vi "PhotonCamera_GetLatestResult.vi"(6 "EstimatedDataAndSampleLatency (Sec)":dbl=0.05 format="%#_13g", 8 "Pass_Through_Time":dbl=-1.0 format="%33.4f", 11 "CameraName":string) -> (1 "HasTargets":bool, 3 "PipelineResult":T1 {"Targets"."AltCameraToTarget"."TRANSLATION3D"."Z" format="%14.3f"; "Targets"."AltCameraToTarget"."TRANSLATION3D"."Y" format="%14.3f"; "Targets"."AltCameraToTarget"."TRANSLATION3D"."X" format="%14.3f"; "Targets"."BestCameraToTarget"."TRANSLATION3D"."Z" format="%14.3f"; "Targets"."BestCameraToTarget"."TRANSLATION3D"."Y" format="%14.3f"; "Targets"."BestCameraToTarget"."TRANSLATION3D"."X" format="%14.3f"})   [LabVIEW 2019, in "PhotonVisionLib.lvlib"]
doc: "Returns the latest pipeline result.\n\nInputs:\n - cameraName -- The nickname of the camera (found in the PhotonVision UI).\n - PassThroughTime -- (Optional. Default: Use FPGA time.) Time. Once time is available from network tables, this won't be needed. (Seconds)\n - EstimatedDataAndSampleLatency -- Estimated Network Table packet latency. This is based on the frames per second and other communications latencies. (Optional. Default: 0.050) Once time is available from network tables, this won't be needed. \n\nOutputs:\n - PipelineResult -- The latest pipeline result data cluster\n - HasTargets -- Boolean indicating if any targets were found"
uses:
  PhotonVisionLib.lvlib
  TypeDef/PhotonPipelineResultType.ctl
  TypeDef/PhotonTrackedTargetType.ctl
  TypeDef/TargetCornerType.ctl
  <vilib>/Rock Robotics/WPI/ThirdParty/JAS_Junk/TrajLib/TypeDef/TRANSFORM3D.ctl
  <vilib>/Rock Robotics/WPI/ThirdParty/JAS_Junk/TrajLib/TypeDef/TRANSLATION3D.ctl
  <vilib>/Rock Robotics/WPI/ThirdParty/JAS_Junk/TrajLib/TypeDef/ROTATION3D.ctl
  <vilib>/Rock Robotics/WPI/ThirdParty/JAS_Junk/TrajLib/TypeDef/QUATERNION.ctl
  Packet_decode_Flt64.vi
  Packet_decode_ByteI8.vi
  PhotonTrackedTarget_CreateFromPacket.vi
  TargetCorner_New.vi
  Packet_decode_Int32.vi
  Packet_decode_Transform3d.vi
  <vilib>/Rock Robotics/WPI/ThirdParty/JAS_Junk/TrajLib/VI/Transform3d_Create_Trans3dRot3d.vi
  <vilib>/Rock Robotics/WPI/ThirdParty/JAS_Junk/TrajLib/VI/Translation3d_Create.vi
  <vilib>/Rock Robotics/WPI/ThirdParty/JAS_Junk/TrajLib/VI/Rotation3d_Create_Quaternion.vi
  <vilib>/Rock Robotics/WPI/ThirdParty/JAS_Junk/TrajLib/VI/Quaternion_New.vi
  <vilib>/Rock Robotics/WPI/ThirdParty/JAS_Junk/TrajLib/VI/Quaternion_Normalize.vi
  <vilib>/Rock Robotics/WPI/ThirdParty/JAS_Junk/TrajLib/VI/Quaternion_New_Default.vi
  <vilib>/Rock Robotics/Network Tables/NT Read Raw.vi
  <vilib>/Rock Robotics/WPI/ThirdParty/JAS_Junk/TrajLib/Trajectory_Library.lvlib
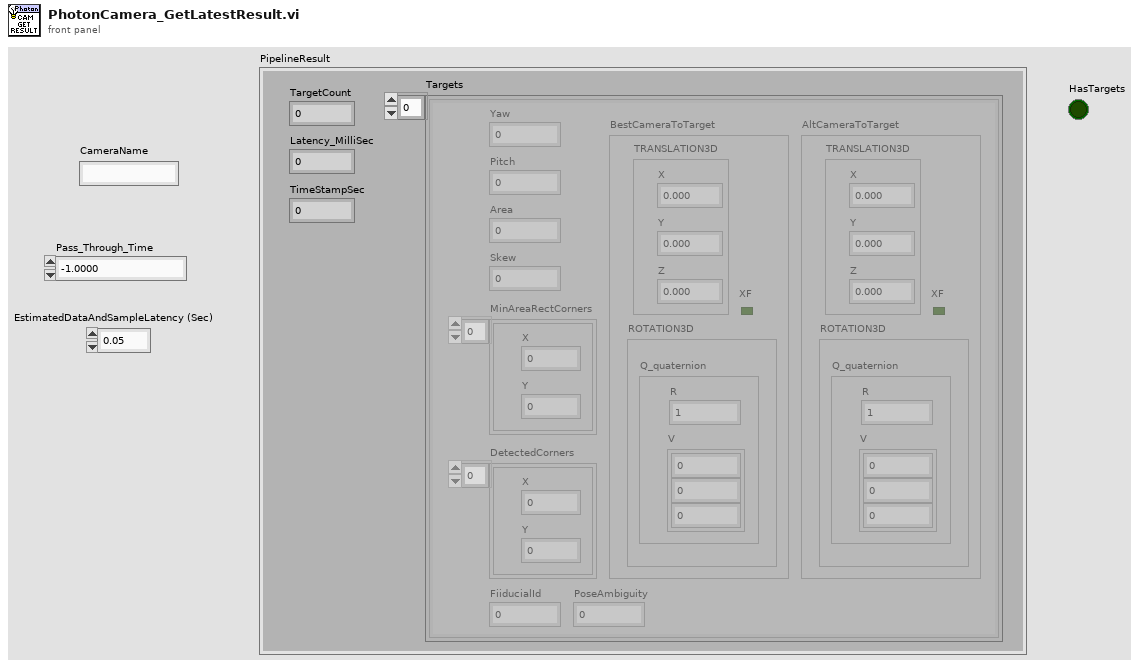
[diagram p1: front panel]
types:
  T1 = typedef "PhotonVisionLib.lvlib/PhotonPipelineResultType.ctl" = cluster{"TargetCount":i32, "Latency_MilliSec":dbl, "Targets":T2[], "TimeStampSec":dbl}
  T2 = typedef "PhotonVisionLib.lvlib/PhotonTrackedTargetType.ctl" = cluster{"Yaw":dbl, "Pitch":dbl, "Area":dbl, "Skew":dbl, "MinAreaRectCorners":T3[], "BestCameraToTarget":T4, "FiiducialId":i32, "AltCameraToTarget":T4, "PoseAmbiguity":dbl, "DetectedCorners":T3[]}
  T3 = typedef "PhotonVisionLib.lvlib/TargetCornerType.ctl" = cluster{"X":dbl, "Y":dbl}
  T4 = typedef "Trajectory_Library.lvlib/TRANSFORM3D.ctl" = cluster{"TRANSLATION3D":T5, "ROTATION3D":T6, "XF":bool}
  T5 = typedef "Trajectory_Library.lvlib/TRANSLATION3D.ctl" = cluster{"X":dbl, "Y":dbl, "Z":dbl}
  T6 = typedef "Trajectory_Library.lvlib/ROTATION3D.ctl" = cluster{"Q_quaternion":T7}
  T7 = typedef "Trajectory_Library.lvlib/QUATERNION.ctl" = cluster{"R":dbl, "V":dbl[]}
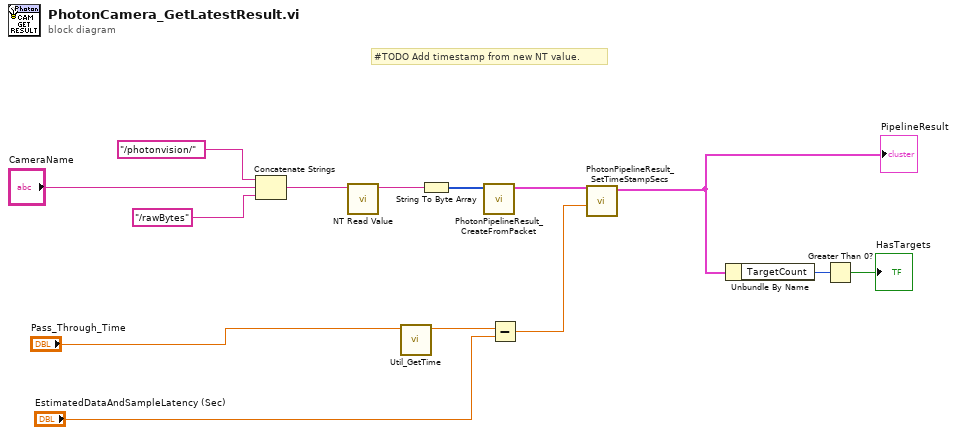
[diagram p0: block diagram]
diagram:
  # "#TODO Add timestamp from new NT value."
  n1 = Concatenate Strings("/photonvision/", "CameraName", "/rawBytes") -> (w11:string)
  n2 = call-poly <vilib>:"NT Read Value.vi"("Name"=w11) -> ("Raw"=w10:string)  [unwired: 9 in, 1 out]
  n3 = call <vilib>:"Util_GetTime.vi"("Pass_Through_Time"="Pass_Through_Time") -> ("FPGA_Time_Seconds"=w3:dbl)  [unwired: 8 in, 2 out]
  n4 = String To Byte Array(string=w10) -> (unsigned byte array=w9:u8[])
  n5 = call "PhotonPipelineResult_CreateFromPacket.vi"("RawData"=w9) -> ("PhotonPipelineResult"=w6:T1)  [unwired: 10 in]
  n6 = Subtract(x=w3, y="EstimatedDataAndSampleLatency (Sec)") -> (x-y=w2:dbl)
  n7 = call "PhotonPipelineResult_SetTimeStampSecs.vi"("TimeStampSec"=w2, "PhotonPipelineResult"=w6) -> ("Out PhotonPipelineResult"=w5:T1)  [unwired: 9 in]
  "PipelineResult" <- w5
  n8 = Unbundle By Name(w5) -> ("TargetCount"=w8:i32)
  n9 = Greater Than 0?(x=w8) -> (x > 0?=→"HasTargets":bool)
